vi "Get Channel.vi"(8 "error in (no error)":errorcluster, 10 "Channel":T2=enum."Channel 2", 11 "VISA Refnum in":refnum<visa-resource-name>="COM1") -> (0 "error out":errorcluster, 2 "Channel Parameters":T1, 3 "VISA Refnum out":refnum<visa-resource-name>)   [LabVIEW 2019, in "KH7008.lvlib"]
uses:
  KH7008.lvlib
  typedefs/Channel--Enum.ctl
  typedefs/SetAll--Cluster.ctl
  typedefs/Gain--Enum.ctl
  typedefs/Input Configuration--Enum.ctl
  typedefs/Shunt--Enum.ctl
  typedefs/Coupling--Enum.ctl
  typedefs/Filter--Enum.ctl
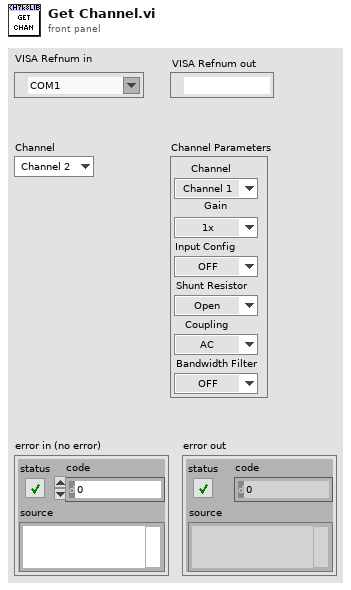
[diagram p1: front panel]
types:
  T1 = typedef "KH7008.lvlib/SetAll--Cluster.ctl" = cluster{"Channel":T2, "Gain":T3, "Input Config":T4, "Shunt Resistor":T5, "Coupling":T6, "Bandwidth Filter":T7}
  T2 = typedef "KH7008.lvlib/Channel--Enum.ctl" = enum8{"Channel 1", "Channel 2", "Channel 3", "Channel 4", "Channel 5", "Channel 6", "Channel 7", "Channel 8"}
  T3 = typedef "KH7008.lvlib/Gain--Enum.ctl" = enum8{"1x", "10x", "100x", "1000x"}
  T4 = typedef "KH7008.lvlib/Input Configuration--Enum.ctl" = enum8{"OFF", "SE+", "SE-", "DIFF"}
  T5 = typedef "KH7008.lvlib/Shunt--Enum.ctl" = enum8{"Open", "50 Ohms", "500 Ohms", "5k Ohms", "50k Ohms", "10M Ohm"}
  T6 = typedef "KH7008.lvlib/Coupling--Enum.ctl" = enum8{"AC", "DC"}
  T7 = typedef "KH7008.lvlib/Filter--Enum.ctl" = enum8{"OFF", "ON"}
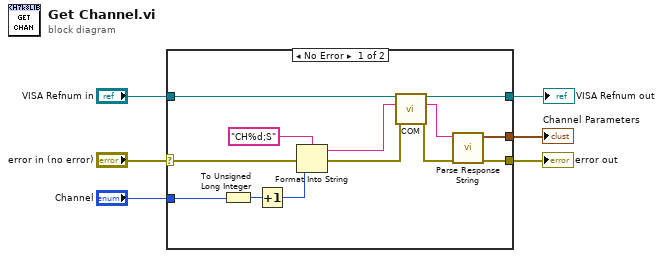
[diagram p0: block diagram]
diagram:
  n1 = case shown="No Error" "error in (no error)" {
    selector: "error in (no error)" -> [w14 w21]
    tunnel: [w18 w21] -> w6
    tunnel: [w16 _] -> w5
    tunnel: "Channel" -> [w15 _]
    tunnel: [w11 w20] -> w2
    tunnel: "VISA Refnum in" -> [w10 w20]
    frame No Error {
      n2 = To Unsigned Long Integer(number=w15) -> (unsigned 32bit integer=w7:u32)
      n3 = Increment(x=w7) -> (x+1=w8:u32)
      n4 = Format Into String(format string="CH%d;S", error in=w14, w8) -> (resulting string=w12:string, error out=w13:errorcluster)  [unwired: 1 in]
      n5 = call "COM.vi"("error in (no error)"=w13, "Command"=w12, "VISA Refnum in"=w10) -> ("error out"=w19:errorcluster, "Response"=w17:string, "VISA Refnum out"=w11:refnum<visa-resource-name>)  [unwired: 6 in]
      n6 = call "Parse Response String.vi"("error in (no error)"=w19, "Response String"=w17) -> ("error out"=w18:errorcluster, "Channel Parameters"=w16:T1)  [unwired: 8 in]
    }
    frame Error {
    }
  }
  "error out" <- w6
  "VISA Refnum out" <- w2
  "Channel Parameters" <- w5
